vi "From MsgPack bytes.vi"(8 "error in (no error)":errorcluster, 11 "bytes":u8[](array[numeric]) format="%x") -> (0 "error out":errorcluster, 3 "MsgPackArray out":refnum<class "MsgPackArray.lvclass">)   [LabVIEW 2020, in "wamplv.lvlib" / "MsgPackArray.lvclass"]
uses:
  MsgPackArray.lvclass
  MsgPackArray.lvclass/MsgPackArray.ctl
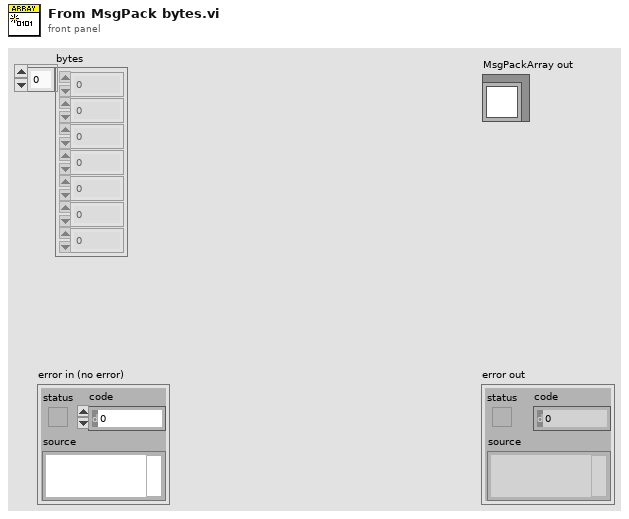
[diagram p1: front panel]
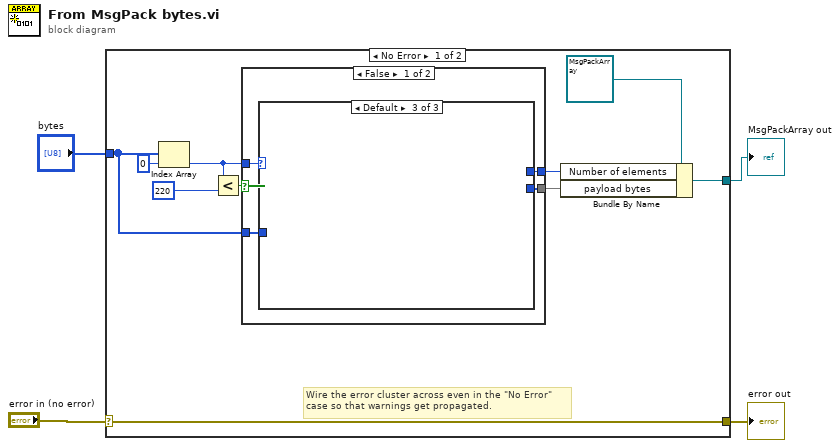
[diagram p0: block diagram]
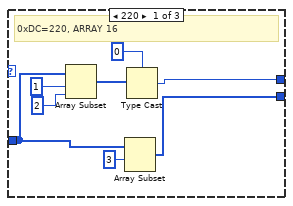
[diagram p2: hidden frame]
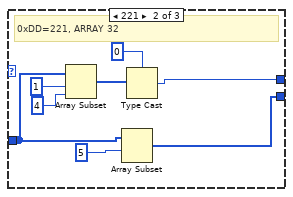
[diagram p3: hidden frame]
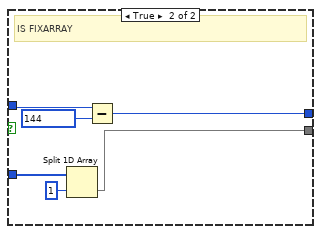
[diagram p4: hidden frame]
diagram:
  n1 = case shown="No Error" "error in (no error)" {
    selector: "error in (no error)" -> [w14 w41]
    tunnel: [w14 w41] -> w3
    tunnel: "bytes" -> [w7 _]
    tunnel: [w5 _] -> w1
    frame No Error {
      # "Wire the error cluster across even in the \"No Error\"\ncase so that warnings get propagated."
      n2 = Index Array(array=w7, index=0) -> (element=w10:u8)
      n3 = Less?(x=w10, y=u8 220) -> (x < y?=w11:bool)
      n4 = case shown="False" w11 {
        tunnel: w10 -> [w18 w40]
        tunnel: [w16 w38] -> w8
        tunnel: w7 -> [w17 w37]
        tunnel: [w15 w35] -> w6
        frame False {
          n5 = case shown="Default" w18 {
            tunnel: w17 -> [w21 w29 _]
            tunnel: [w22 w30 _] -> w16
            tunnel: [w20 w27 _] -> w15
            frame 220 {
              # "0xDC=220, ARRAY 16"
              n6 = Array Subset(array=w21, index=1, length=2) -> (w24:u8[])
              n7 = Array Subset(array=w21, index=3) -> (w20:u8[])  [unwired: 1 in]
              n8 = Type Cast(type=u16 0, x=w24) -> (*(type *) &x=w22:u16)
            }
            frame 221 {
              # "0xDD=221, ARRAY 32"
              n9 = Array Subset(array=w29, index=1, length=4) -> (w32:u8[])
              n10 = Array Subset(array=w29, index=5) -> (w27:u8[])  [unwired: 1 in]
              n11 = Type Cast(type=u32 0, x=w32) -> (*(type *) &x=w30:u32)
            }
            frame Default {
            }
          }
        }
        frame True {
          # "IS FIXARRAY"
          n12 = Split 1D Array(array=w37, index=1) -> (second subarray=w35:u8[])  [unwired: 1 out]
          n13 = Subtract(x=w40, y=u8 144) -> (x-y=w38:u8)
        }
      }
      n14 = Bundle By Name(cluster=refnum<class "MsgPackArray.lvclass"> refnum ("wamplv.lvlib:MsgPackArray.lvclass"), "Number of elements"=w8, "payload bytes"=w6) -> (w5:refnum<class "MsgPackArray.lvclass">)
    }
    frame Error {
    }
  }
  "error out" <- w3
  "MsgPackArray out" <- w1
